vi "ms time string to LV timestamp.vi"(11 "String":string) -> (3 "Time Stamp":timestamp)   [LabVIEW 2020]
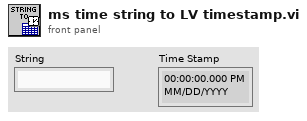
[diagram p1: front panel]
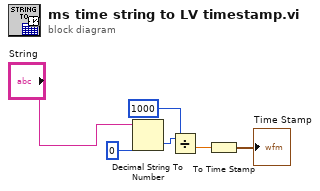
[diagram p0: block diagram]
diagram:
  n1 = Decimal String To Number(string="String", default (0L)=i64 0 ("default (0 I32)")) -> (number=w3:i64)  [unwired: 1 in, 1 out]
  n2 = Divide(x=w3, y=i64 1000) -> (x/y=w5:dbl)
  n3 = To Time Stamp(1:w5) -> (0:→"Time Stamp":timestamp)
